vi "拆解cluster到最後.vi"(11 "Clust Refnum":refnum<vi>) -> (3 "Array":bool[](array[boolean]))   [LabVIEW 2015]
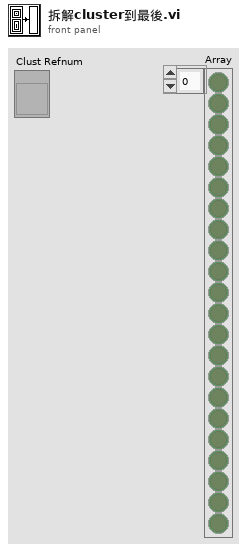
[diagram p1: front panel]
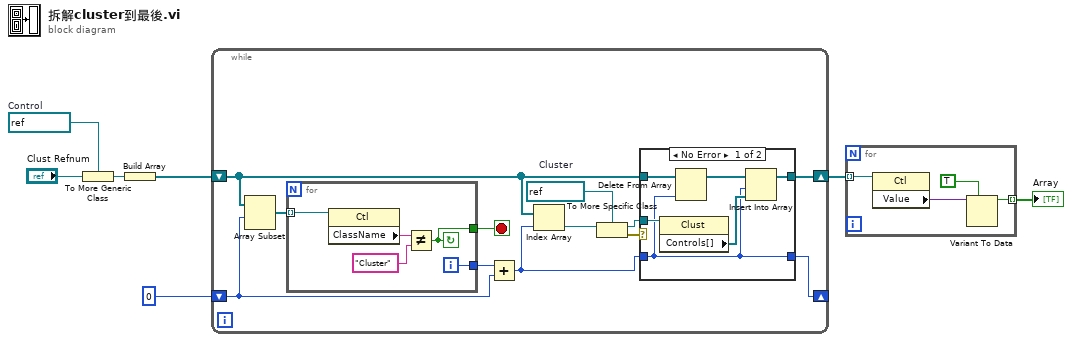
[diagram p0: block diagram]
diagram:
  w6 = refnum<vi> refnum  # Control
  n1 = To More Generic Class(target class=w6, reference="Clust Refnum") -> (generic class reference=w7:refnum<vi>)
  n2 = Build Array(w7) -> (w5:refnum<vi>[])
  n3 = while {
    shift-right: [w18] -> w2
    shift-left: w5 -> [w13]
    shift-right: [w19] -> _
    shift-left: 0 -> [w14]
    stop <- w16 stop-if-true
    w11 = refnum<vi> refnum  # Cluster
    n4 = Array Subset(array=w13, index=w14) -> (w17:refnum<vi>[])  [unwired: 1 in]
    n5 = for {
      tunnel: w17 -> [w32] mode=indexing
      tunnel: [w29] -> w16
      tunnel: [w28] -> w15
      i -> [w28]
      stop <- w29 continue-if-true
      n6 = property class="Ctl"(reference=w32) -> ("ClassName"=w31:string)  [unwired: 1 in, 2 out]
      n7 = Not Equal?(x=w31, y="Cluster") -> (x != y?=w29:bool)
    }
    n8 = Add(x=w15, y=w14) -> (x+y=w8:i32)
    n9 = Index Array(array=w13, index=w8) -> (element=w12:refnum<vi>)
    n10 = To More Specific Class(target class=w11, reference=w12) -> (specific class reference=w9:refnum<vi>, error out=w10:errorcluster)  [unwired: 1 in]
    n11 = case shown="No Error" w10 {
      tunnel: w13 -> [w25 w27]
      tunnel: w8 -> [w20 w26]
      tunnel: w9 -> [w23 _]
      tunnel: [w21 w27] -> w18
      tunnel: [w20 w26] -> w19
      frame No Error {
        n12 = property class="Clust"(reference=w23) -> ("Controls[]"=w22:refnum<vi>[])  [unwired: 1 in, 2 out]
        n13 = Delete From Array(array=w25, index=w20) -> (array with subset deleted=w24:refnum<vi>[])  [unwired: 1 in, 1 out]
        n14 = Insert Into Array(array=w24, index=w20, new element=w22) -> (w21:refnum<vi>[])
      }
      frame Error {
      }
    }
  }
  n15 = for {
    tunnel: w2 -> [w36] mode=indexing
    tunnel: [w33] -> w4 mode=indexing
    n16 = property class="Ctl"(reference=w36) -> ("Value"=w35:variant)  [unwired: 1 in, 2 out]
    n17 = Variant To Data(type=TRUE, Variant=w35) -> (data=w33:bool)  [unwired: 1 in, 1 out]
  }
  "Array" <- w4
